vi "FGV Usage.vi"() -> ()   [LabVIEW 2024]
panel:
  in  "stop":bool
  in  "C":dbl
  in  "B":bool
  in  "A":bool
  in  "D":dbl
  out "y 2":dbl
  out "y":bool
  # "Overview:\nIn this VI, Global variables are used from different variables. \nWhen a variable is used for mutiple times we go for global variables where value for it is given by declaring it in the new VI and saved.\nwe can select that whenever there is a need."
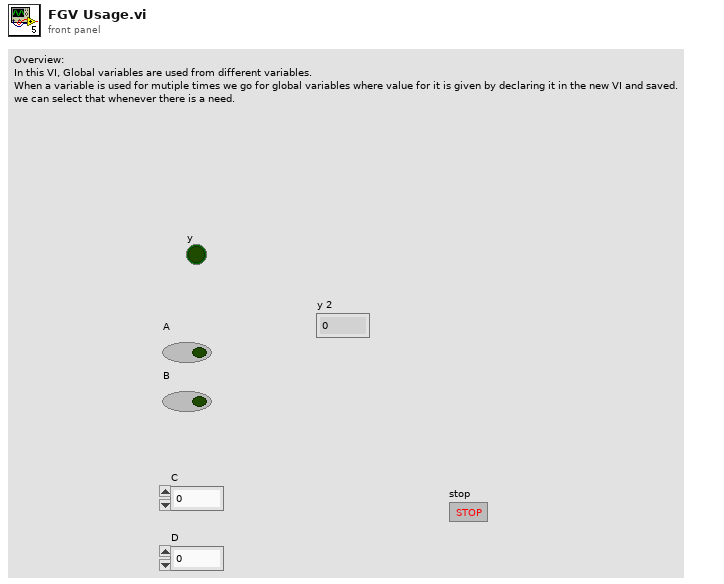
[diagram p1: front panel]
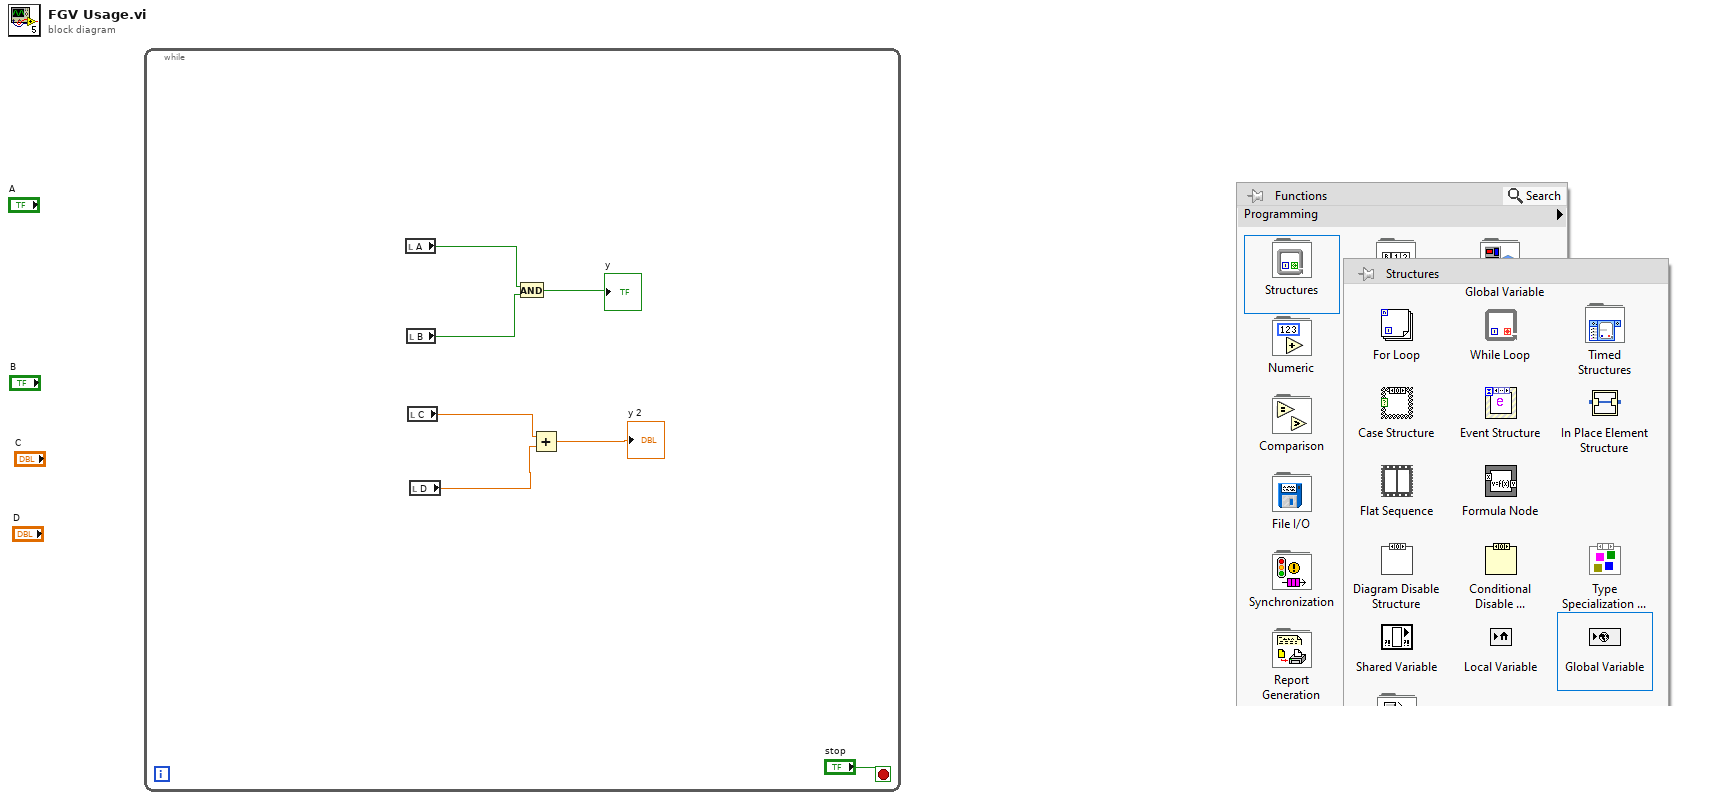
[diagram p0: block diagram]
diagram:
  n1 = while {
    stop <- "stop" stop-if-true
    n2 = local read "A"() -> (w6:bool)
    n3 = local read "B"() -> (w5:bool)
    n4 = local read "C"() -> (w3:dbl)
    n5 = local read "D"() -> (w2:dbl)
    n6 = And(x=w6, y=w5) -> (x .and. y?=→"y":bool)
    n7 = Add(x=w3, y=w2) -> (x+y=→"y 2":dbl)
  }
